vi "get and log info.vi"(8 "error in":errorcluster, 10 "log data?":bool, 11 "Teensy Serial Port":refnum<visa-resource-name>) -> (0 "error out":errorcluster, 2 "info":T1, 3 "LADY GAGA v2 Serial Port out":refnum<visa-resource-name>)   [LabVIEW 2013]
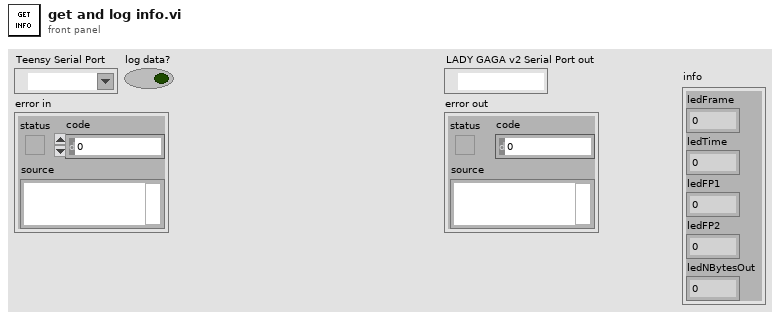
[diagram p1: front panel]
types:
  T1 = cluster{"ledFrame":i32, "ledTime":i32, "ledFP1":i32, "ledFP2":i32, "ledNBytesOut":i32}
  T2 = enum16{"R - open file for Reading", "W - open file for Writing", "S - send bytes", "F - fetch bytes", "B - begin experiment", "E - end experiment", "N - set number of bits per frame", "I - get info", "Q - Quiet (only error msgs)", "L - Loud (acknowledge all)", "T - set stimulus state", "Y - ready to start experiment", "H - useless Help message"}
  T3 = enum16{"Reset Table", "Get Values", "Add Value", "Get Table", "Get Spreadsheet", "set stack writer"}
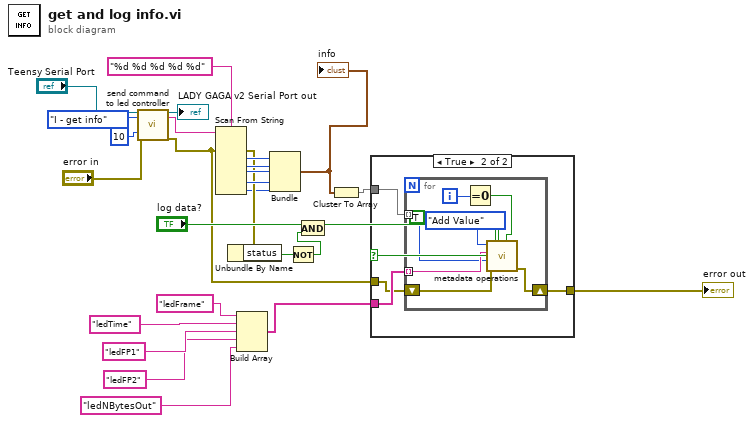
[diagram p0: block diagram]
diagram:
  n1 = call "send command to led controller.vi"("Teensy Serial Port"="Teensy Serial Port", "Command"=T2."I - get info", "milliseconds to wait between write and read"=u32 10, "error in"="error in") -> ("teensy serial port out"=→"LADY GAGA v2 Serial Port out":refnum<visa-resource-name>, "response"=w25:string, "error out"=w8:errorcluster)  [unwired: 10 in, 3 out]
  n2 = Scan From String(format string="%d %d %d %d %d", input string=w25, error in=w8) -> (error out=w7:errorcluster, output 1=w20:i32, output 2=w19:i32, output 3=w18:i32, output 4=w17:i32, output 5=w3:i32)  [unwired: 6 in, 2 out]
  n3 = Unbundle By Name(w7) -> ("status"=w6:bool)
  n4 = Build Array("ledFrame", "ledTime" ("element"), "ledFP1" ("element"), "ledFP2" ("element"), "ledNBytesOut" ("element")) -> (w10:string[])
  n5 = Bundle(w20, w19, w18, w17, w3) -> (w15:cluster{i32, i32, i32, i32, i32})  [unwired: 1 in]
  "info" <- w15
  n6 = Not(x=w6) -> (.not. x?=w4:bool)
  n7 = And(x="log data?", y=w4) -> (x .and. y?=w5:bool)
  n8 = Cluster To Array(cluster=w15) -> (array=w11:i32[])
  n9 = case shown="True" w5 {
    tunnel: w11 -> [_ w32]
    tunnel: w10 -> [_ w31]
    tunnel: w8 -> [w28 w30]
    tunnel: [w28 w29] -> w9
    frame False {
    }
    frame True {
      n10 = for {
        tunnel: w32 -> [w35] mode=indexing
        tunnel: w31 -> [w36] mode=indexing
        shift-right: [w33] -> w29
        shift-left: w30 -> [w34]
        i -> [w39]
        n11 = Equal To 0?(x=w39) -> (x = 0?=w38:bool)
        n12 = call "metadata operations.vi"("add time?"=w38, "add to stack writer"=TRUE, "error in (no error)"=w34, "value"=w35, "key"=w36, "Operation"=T3."Add Value") -> ("error out"=w33:errorcluster)  [unwired: 2 in, 3 out]
      }
    }
  }
  "error out" <- w9
